vi "OldIntakeGlobal.vi"() -> ()   [LabVIEW 2023]
uses:
  OldIntakeState.ctl
panel:
  out "MotorDemand 2":dbl
  out "IntakeDmdValue 2":dbl=0.4
  out "FeedDmdValue":dbl=0.8
  out "SpitOutDmdValue":dbl=-0.2
  out "IntakeDmdValue":dbl=0.4
  out "MotorDemand":dbl
  out "SpeedRPM":dbl
  out "IntakeCurrentState":T1
  out "IntakeSensor":bool
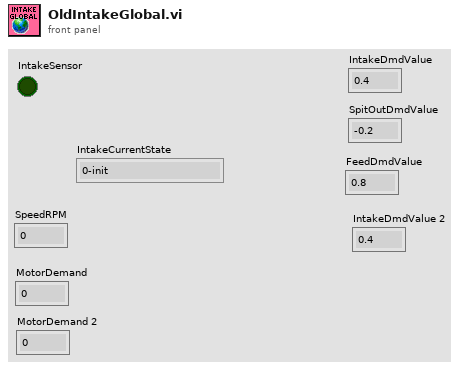
[diagram p1: front panel]
types:
  T1 = typedef "OldIntakeState.ctl" = enum16{"0-init", "1-cancel", "2-wait-for-cmd", "3-intake-check-for-note", "4-intake-start-intake", "5-intake-have-note-yet", "6-intake-stop-motor", "7-spit-out", "8-feed-note-to-shooter"}
diagram:
